vi "Read XML_Parse RTs.vi"(8 "error in (no error)":errorcluster, 10 "channel in":T1, 11 ".NET Refnum in":refnum<k24>) -> (0 "error out":errorcluster, 2 "channel out":T1, 3 ".NET Refnum out":refnum<k24>)   [LabVIEW 2017, in "Ballard 1553 System Explorer.lvlib"]
uses:
  Ballard 1553 System Explorer.lvlib
  Ballard_Channel.ctl
  Ballard_BC.ctl
  Ballard_message.ctl
  Ballard_messageType.ctl
  Ballard_CWD1.ctl
  Ballard_CWD2.ctl
  Ballard_minorFrame.ctl
  Ballard_majorFrame.ctl
  Ballard_acyclicFrame.ctl
  Ballard_RT.ctl
  Ballard_RT subAddress.ctl
  Ballard_RT direction.ctl
  Ballard_RT rtMode.ctl
  Ballard_RT modeCode.ctl
  D:/Ballard-1553-Custom-Device Inline Async/Source/System Explorer/SubVIs/Parse XML Ballard/Ballard_BTI_XML_MIL_STD_1553_Deserializer.dll
  Ballard_BTI_XML_MIL_STD_1553_Deserializer.dll
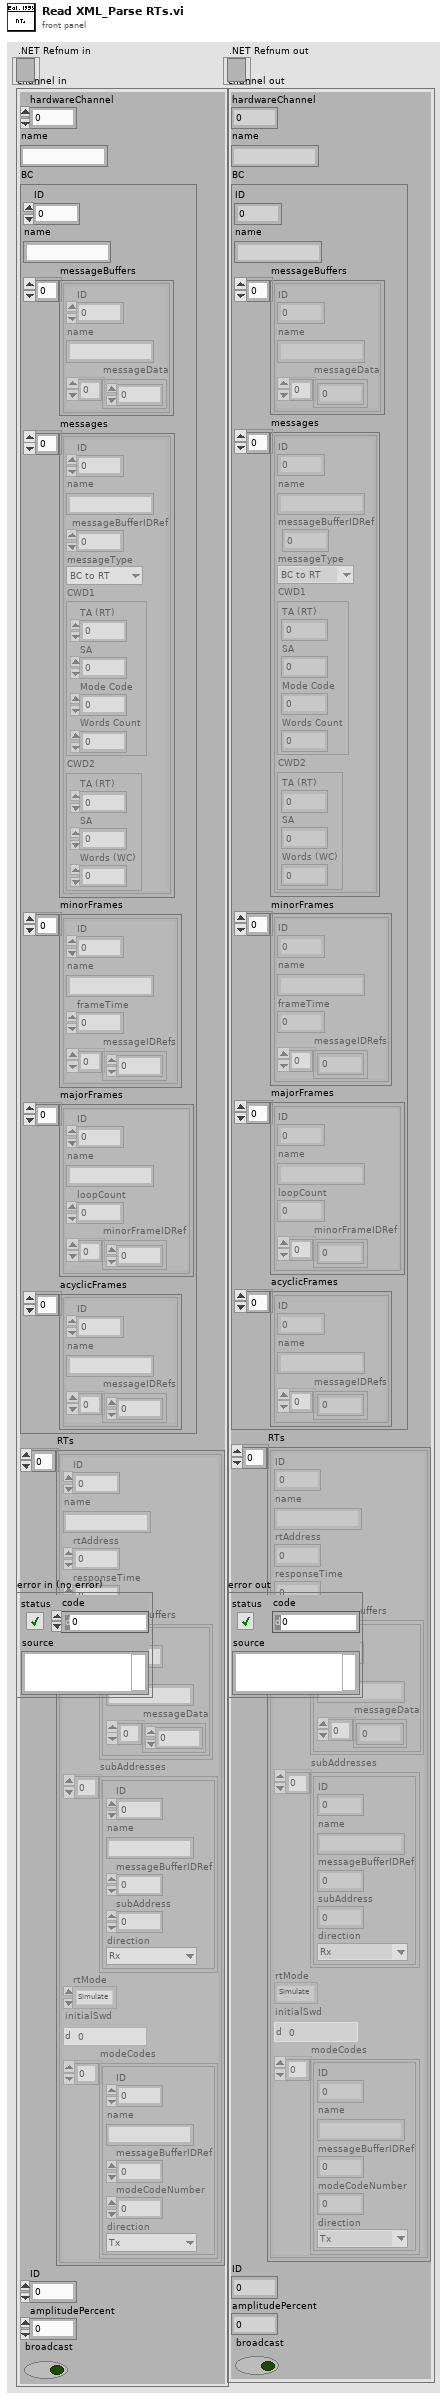
[diagram p1: front panel]
types:
  T1 = typedef "Ballard 1553 System Explorer.lvlib/Ballard_Channel.ctl" = cluster{"hardwareChannel":i32, "name":string, "BC":T2, "RTs":T10[], "ID":i32, "amplitudePercent":dbl, "broadcast":bool}
  T2 = typedef "Ballard 1553 System Explorer.lvlib/Ballard_BC.ctl" = cluster{"ID":i32, "name":string, "messageBuffers":cluster{"ID":i32, "name":string, "messageData":u16[]}[], "messages":T3[], "minorFrames":T7[], "majorFrames":T8[], "acyclicFrames":T9[]}
  T3 = typedef "Ballard 1553 System Explorer.lvlib/Ballard_message.ctl" = cluster{"ID":i32, "name":string, "messageBufferIDRef":i32, "messageType":T4, "CWD1":T5, "CWD2":T6}
  T4 = typedef "Ballard 1553 System Explorer.lvlib/Ballard_messageType.ctl" = enum16{"BC to RT", "RT to BC", "RT to RT", "MC (Rx)", "MC (Tx)"}
  T5 = typedef "Ballard 1553 System Explorer.lvlib/Ballard_CWD1.ctl" = cluster{"TA (RT)":i8, "SA":i8, "Mode Code":i8, "Words Count":i8}
  T6 = typedef "Ballard 1553 System Explorer.lvlib/Ballard_CWD2.ctl" = cluster{"TA (RT)":i8, "SA":i8, "Words (WC)":i8}
  T7 = typedef "Ballard 1553 System Explorer.lvlib/Ballard_minorFrame.ctl" = cluster{"ID":i32, "name":string, "frameTime":i32, "messageIDRefs":i32[]}
  T8 = typedef "Ballard 1553 System Explorer.lvlib/Ballard_majorFrame.ctl" = cluster{"ID":i32, "name":string, "loopCount":i32, "minorFrameIDRef":i32[]}
  T9 = typedef "Ballard 1553 System Explorer.lvlib/Ballard_acyclicFrame.ctl" = cluster{"ID":i32, "name":string, "messageIDRefs":i32[]}
  T10 = typedef "Ballard 1553 System Explorer.lvlib/Ballard_RT.ctl" = cluster{"ID":i32, "name":string, "rtAddress":i8, "responseTime":i32, "messageBuffers":cluster{"ID":i32, "name":string, "messageData":u16[]}[], "subAddresses":T11[], "rtMode":T13, "initialSwd":u16, "modeCodes":T14[]}
  T11 = typedef "Ballard 1553 System Explorer.lvlib/Ballard_RT subAddress.ctl" = cluster{"ID":i32, "name":string, "messageBufferIDRef":i32, "subAddress":i8, "direction":T12}
  T12 = typedef "Ballard 1553 System Explorer.lvlib/Ballard_RT direction.ctl" = enum16{"Tx", "Rx"}
  T13 = typedef "Ballard 1553 System Explorer.lvlib/Ballard_RT rtMode.ctl" = enum16{"Simulate", "Monitor", "Disable"}
  T14 = typedef "Ballard 1553 System Explorer.lvlib/Ballard_RT modeCode.ctl" = cluster{"ID":i32, "name":string, "messageBufferIDRef":i32, "modeCodeNumber":i8, "direction":T12}
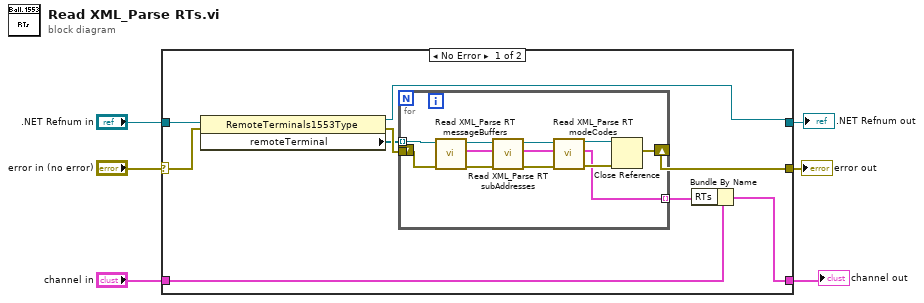
[diagram p0: block diagram]
diagram:
  n1 = case shown="No Error" "error in (no error)" {
    selector: "error in (no error)" -> [w7 w29]
    tunnel: [w15 w28] -> w6
    tunnel: "channel in" -> [w13 w28]
    tunnel: [w12 w29] -> w4
    tunnel: [w10 w30] -> w3
    tunnel: ".NET Refnum in" -> [w8 w30]
    frame No Error {
      n2 = property class="RemoteTerminals1553Type"(reference=w8, error in=w7) -> (reference out=w10:refnum<k24>, error out=w11:errorcluster, "remoteTerminal"=w9:refnum<k24>[])
      n3 = for {
        tunnel: w9 -> [w27] mode=indexing
        tunnel: w11 -> [w26]
        tunnel: [w16] -> w14 mode=indexing
        shift-right: [w25] -> w12
        shift-left: _ -> [_]
        n4 = call "Read XML_Parse RT messageBuffers.vi"("error in (no error)"=w26, "RemoteTerminal1553Type"=w27) -> ("error out"=w23:errorcluster, "RT"=w22:T10, "RemoteTerminal1553Type"=w24:refnum<k24>)  [unwired: 7 in]
        n5 = call "Read XML_Parse RT subAddresses.vi"("error in (no error)"=w23, "RT in"=w22, "RemoteTerminal1553Type"=w24) -> ("error out"=w18:errorcluster, "RT out"=w17:T10, "RemoteTerminal1553Type"=w21:refnum<k24>)  [unwired: 6 in]
        n6 = call "Read XML_Parse RT modeCodes.vi"("error in (no error)"=w18, "RT in"=w17, "RemoteTerminal1553Type"=w21) -> ("error out"=w19:errorcluster, "RT out"=w16:T10, "RemoteTerminal1553Type"=w20:refnum<k24>)  [unwired: 6 in]
        n7 = Close Reference(reference=w20, error in (no error)=w19) -> (error out=w25:errorcluster)
      }
      n8 = Bundle By Name(cluster=w13, "RTs"=w14) -> (w15:T1)
    }
    frame Error {
    }
  }
  "channel out" <- w6
  "error out" <- w4
  ".NET Refnum out" <- w3
